vi "InitScope5782_six_channel.vi"(6 "FpgaRef5782":refnum<class "FpgaRefx410.lvclass">, 8 "error in (no error)":errorcluster, 10 "FpgaRef5761":refnum<class "FpgaRef5761.lvclass">, 11 "Scope5785_six_channel":refnum<class "Scope5782_six_channel.lvclass">) -> (0 "error out":errorcluster, 3 "Scope5785_six_channel out":refnum<class "Scope5782_six_channel.lvclass">)   [LabVIEW 2025, in "Scope5782_six_channel.lvclass"]
uses:
  Scope5782_six_channel.lvclass
  FpgaRef/FpgaRef5761/FpgaRef5761.lvclass
  FpgaRef/FpgaRefx410/FpgaRefx410.lvclass
  FPGA/fpga_settings.ctl
  Scope5782_six_channel.lvclass/Scope5782_six_channel.ctl
  <vilib>/rvi/FXPMathLib/FxpInterpret/XNode/nifxpmath_Interpret.xnode
  FpgaRef/FpgaRefBase/FpgaRefBase.lvclass
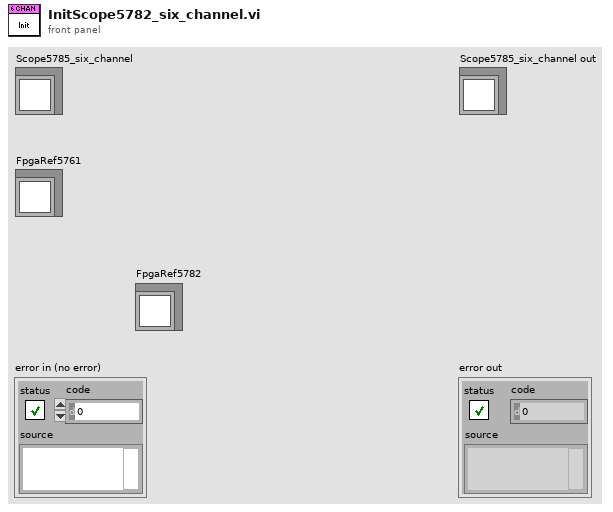
[diagram p1: front panel]
types:
  T1 = typedef "fpga_settings.ctl" = enum16{"Feedback Enable", "New FIR coeffs", "FIR shift", "Enable filter", "Set Downsample", "Downsample", "CIC Gain", "Record length", "Trigger samples", "Quiet time", "a_am", "b_am", "Use fixed delay", "fixed sin_fi", "fixed cos_fi", "Ki*Tau", "Kp", "Kd_Tau", "Fi_start", "Fi_delta", "DC_offs 0", "DC_offs 1", "DC_offs 2", "DC_offs 3", "Ki*Tau am", "Kp am", "Kd_Tau am", "Feedback AM", "Trigger delay", "Feedback delay", "Setpoint enable", "Beam enable", "Samples to acquire", "Cavity Enable", "Cavity C1", "Cavity C2", "Cavity C3", "Cavity C4", "Cavity C5", "Input delay", "Ki*Tau Q", "Kp Q", "Kd_Tau Q", "Adaptive FF enable", "Feedforward a0", "Feedforward b0", "FF src adress", "FF dest adress", "Output scale", "Input scale", "Host scale", "FF_IIR b0", "FF_IIR b1", "FF_IIR b2", "FF_IIR-a1", "FF_IIR-a2", "Enable HW trigger", "Virtual cavity", "Samples to skip", "Samples to skip 2", "Samples to skip 3", "Cavity C3_2", "Cavity C4_2", "Cavity C5_2", "Cavity C3_3", "Cavity C4_3", "Cavity C5_3", "Cavity_w0_dt", "Piezo setting", "Quench t0", "Quench tau set", "Quench enabled", "Quench reset", "PID enabled I", "PID enabled Q", "Cavity filter a", "Cavity filter b", "Disable e(n)", "FF e(n) src address", "FF first address", "FF last address", "FF PID first address", "FF PID last address", "Amp IIR b0", "Amp IIR b1", "Amp IIR b2", "Amp IIR-a1", "Amp IIR-a2", "Adaptation factor", "Inv Amp LP b0", "Inv Amp LP b1", "Inv Amp LP b2", "Inv Amp LP-a1", "Inv Amp LP-a2", "Inv Amp c0", "Inv Amp c1", "Inv Amp c2", "Inv Amp c3", "Inv Amp c4", "Inv Amp -d1", "Inv Amp -d2", "Inv Amp -d3", "Inv Amp -d4", "w12_a", "w12_b", "w12_dt", "w12_scale", "dw_scale", "Extra output select", "Extra fi sin", "Extra fi cos", "Extra output scale", "Quench max output"}
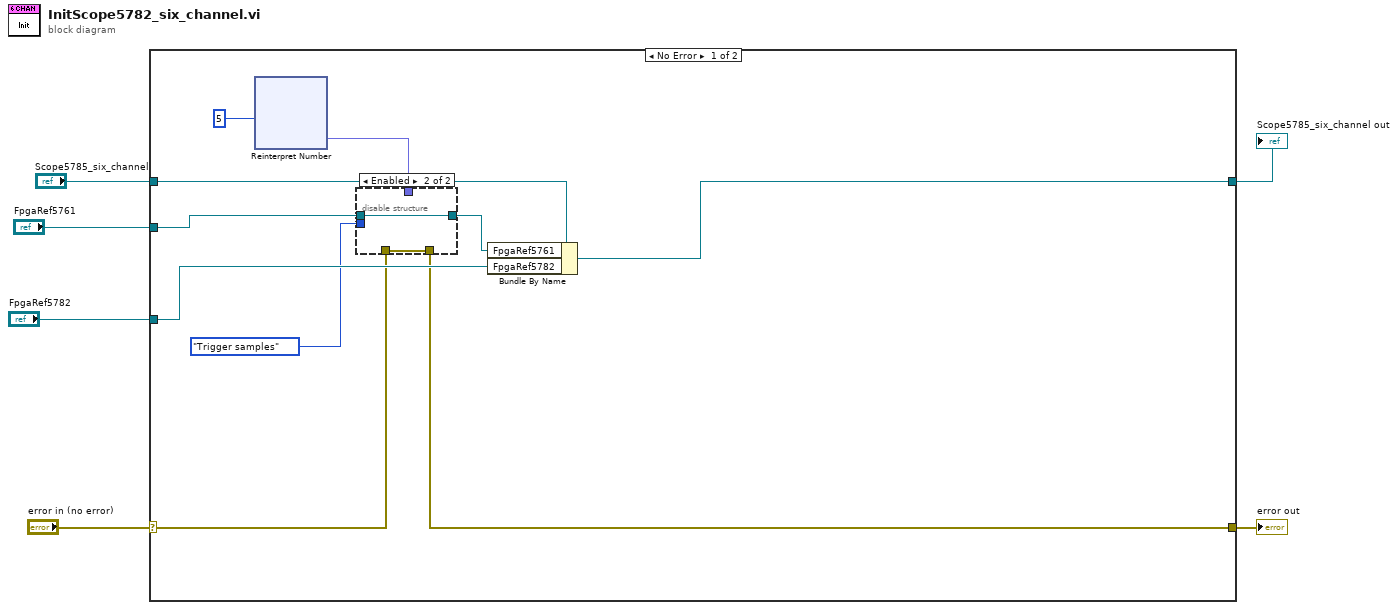
[diagram p0: block diagram]
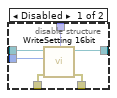
[diagram p2: hidden frame]
diagram:
  n1 = case shown="No Error" "error in (no error)" {
    selector: "error in (no error)" -> [w8 w26]
    tunnel: [w7 w26] -> w5
    tunnel: "Scope5785_six_channel" -> [w16 w25]
    tunnel: "FpgaRef5761" -> [w13 _]
    tunnel: [w15 w25] -> w2
    tunnel: "FpgaRef5782" -> [w14 _]
    frame No Error {
      n2 = xnode "Reinterpret Number"("x"=u16 5 ("trigger samples")) -> ("y"=w10:fxp<+,16,16>)
      n3 = disable-structure shown="Enabled" {
        disable-tunnel: w13 -> [w22 w24]
        disable-tunnel: [w21 w24] -> w12
        disable-tunnel: w10 -> [w20 _]
        disable-tunnel: fpga_settings."Trigger samples" ("FPGA Setting") -> [w19 _]
        disable-tunnel: w8 -> [w18 w23]
        disable-tunnel: [w17 w23] -> w7
        frame Disabled {
          n4 = call "WriteSetting 16bit.vi"("value"=w20, "error in (no error)"=w18, "FPGA Setting"=w19, "FpgaRefBase in"=w22) -> ("error out"=w17:errorcluster, "FpgaRefBase out"=w21:refnum<class "FpgaRef5761.lvclass">)  [unwired: 6 in]
        }
        frame Enabled {
        }
      }
      n5 = Bundle By Name(cluster=w16, "FpgaRef5761"=w12, "FpgaRef5782"=w14) -> (w15:refnum<class "Scope5782_six_channel.lvclass">)
    }
    frame Error {
    }
  }
  "error out" <- w5
  "Scope5785_six_channel out" <- w2
